vi "FTW-Connector-Ask.vi"(0 "FTW Actor Connector":refnum<data-value>, 5 "Request":string, 7 "Receive Timeout":i32=100 format="%dmsec", 9 "Send Timeout":i32 format="%dmsec", 11 "error in":errorcluster) -> (4 "FTW Actor Connector out":refnum<data-value>, 6 "Response":string, 8 "Roundtrip Time":dbl format="%.4psec", 15 "error out":errorcluster)   [LabVIEW 2014]
uses:
  core/FTW-Connector-Core-Type.ctl
  error/FTW-ERR-ThrowError.vi
  error/FTW-ERR-NoErrorConstant.vi
  error/FTW-ERR-CallChain.vi
  string/FTW-STR-ReplaceWhitespace.vi
  json/core/FTW-JSON-Core-EncodingFlags.vi
  reflection/FTW-Reflection-Type.vi
  codegen/xnode/json/fetch/FTW-JSON-Core-GetFlattenedValue.vi
  codegen/xnode/FTW-JSON-Fetch.xnode
panel:
  # "Inputs"
  # "Outputs"
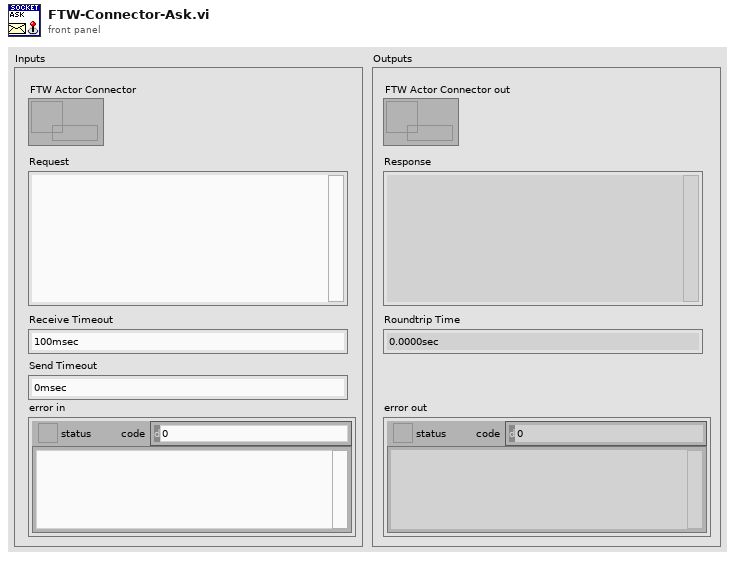
[diagram p1: front panel]
types:
  T1 = typedef "FTW-Connector-Core-Type.ctl" = cluster{"Socket":i64}
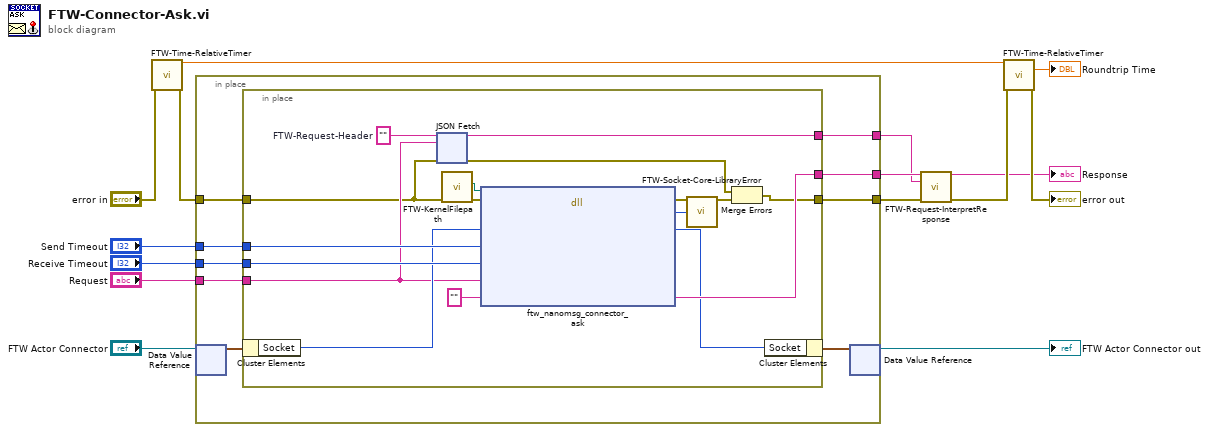
[diagram p0: block diagram]
diagram:
  n1 = call "FTW-Time-RelativeTimer.vi"("error in"="error in") -> ("Current Timer Value"=w8:dbl, "error out"=w9:errorcluster)  [unwired: 12 in, 1 out]
  n2 = in-place {
    in-place-border: w9 -> [w24]
    in-place-border: [w23] -> w4
    in-place-border: [w22] -> w2
    in-place-border: "Send Timeout" -> [w21]
    in-place-border: "Receive Timeout" -> [w20]
    in-place-border: "Request" -> [w19]
    in-place-border: [w16] -> w1
    n3 = in-place-dvr #1("FTW Actor Connector") -> (w18:T1)  [unwired: 1 out]
    n4 = in-place {
      in-place-border: w24 -> [w30]
      in-place-border: [w26] -> w23
      in-place-border: [w40] -> w22
      in-place-border: w21 -> [w39]
      in-place-border: w20 -> [w38]
      in-place-border: w19 -> [w31]
      in-place-border: [w25] -> w16
      w29 = ""  # FTW-Request-Header
      n5 = in-place-cluster #2(w18) -> ("Socket"=w35:i64)
      n6 = xnode "JSON Fetch"("Type and Defaults"=w29, "JSON String"=w31, "error in"=w30) -> ("Values"=w25:string, "error out"=w28:errorcluster)  [unwired: 1 in]
      n7 = call "FTW-KernelFilepath.vi"("error in"=w30) -> ("error out"=w33:errorcluster, "Library Filepath"=w32:path)  [unwired: 8 in, 1 out]
      n8 = dll-call lib="?" fn="ftw_nanomsg_connector_ask"(path in=w32, error in=w33, "Socket Handle"=w35, "Send Timeout"=w39, "Recv Timeout"=w38, "Request"=w31, "Response"="") -> (error out=w41:errorcluster, "Return Value"=w37:i64, "Socket Handle"=w34:i64, "Response"=w40:string)  [unwired: 4 in, 1 out]
      n9 = call "FTW-Socket-Core-LibraryError.vi"("error in"=w41, "Return Value"=w37) -> ("error out"=w27:errorcluster)  [unwired: 13 in]
      n10 = Merge Errors(w28, w27) -> (w26:errorcluster)
      n11 = in-place-cluster #2("Socket"=w34) -> (w17:T1)
    }
    n12 = in-place-dvr #1(w17) -> (→"FTW Actor Connector out":refnum<data-value>)  [unwired: 1 out]
  }
  n13 = call "FTW-Request-InterpretResponse.vi"("Raw Request"=w2, "Request Header"=w1, "error in"=w4) -> ("JSON Response"=→"Response":string, "error out"=w5:errorcluster)  [unwired: 11 in]
  n14 = call "FTW-Time-RelativeTimer.vi"("Previous Timer Value"=w8, "error in"=w5) -> ("Elapsed Time"=→"Roundtrip Time":dbl, "error out"=→"error out":errorcluster)  [unwired: 11 in, 1 out]
